vi "1122test.vi"() -> ()   [LabVIEW 2020]
uses:
  <vilib>/Instr/_visa.llb/VISA Configure Serial Port (Instr).vi
  <vilib>/Utility/file.llb/Write Delimited Spreadsheet (string).vi
panel:
  in  "文件\n路径":path=path "C:/Users/Lenovo/Desktop/data.xls"
  out "错误湿度":dbl
  out "错误温度":dbl
  out "错误芯片ID":u32
  out "温度":dbl(graph)
  out "湿度":dbl(graph)
  in  "字节数(9)":u32=9
  out "缓存区":string="23161"
  in  "串口":refnum<visa-resource-name>="COM4"
  in  "串口设置":T1={"流控制 (0:none)"=0, "停止位 (10: 1 bit)"=10, "奇偶校验 (0:none)"=0, "数据比特 (8)"=8, "比特率 (115200)"=115200} {"数据比特 (8)" min=5 max=8 step=1; "奇偶校验 (0:none)" items=["None", "Odd", "Even", "Mark", "Space"]; "流控制 (0:none)" items=["None", "XON/XOFF", "RTS/CTS", "XON/XOFF & RTS/CTS", "DTR/DSR", "XON/XOFF & DTR/DSR"]}
  in  "开关":bool=TRUE
  out "错误输出":cluster{"status":bool, i32, string}={"status"=FALSE, 1073676294, "VISA Read in Untitled 1.vi"}
  # "温湿度实时监测网络系统"
  # "设计人：苏柯宁 指导老师：李劲松"
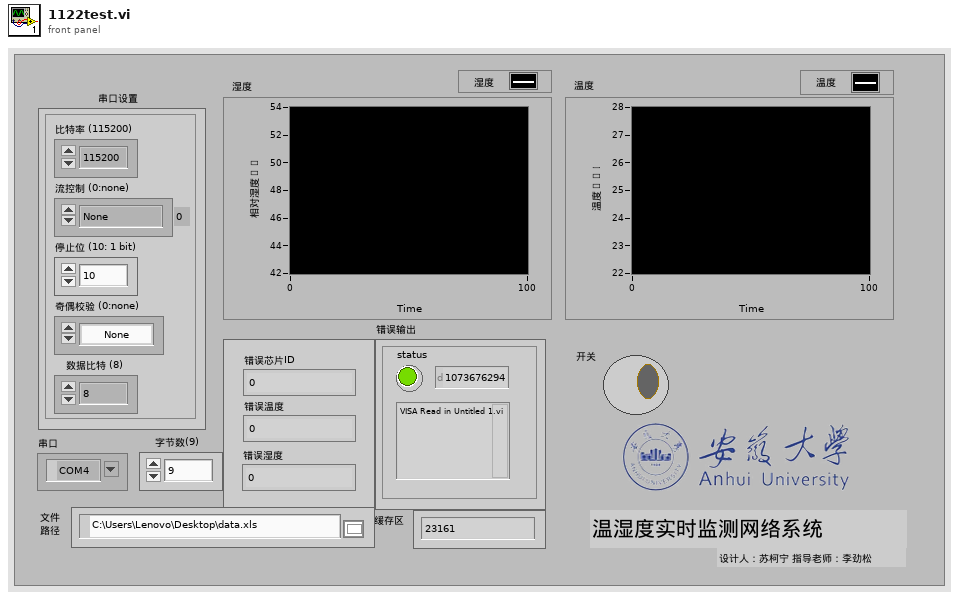
[diagram p1: front panel]
types:
  T1 = cluster{"流控制 (0:none)":u16, "停止位 (10: 1 bit)":u16, "奇偶校验 (0:none)":u16, "数据比特 (8)":u16, "比特率 (115200)":u32}
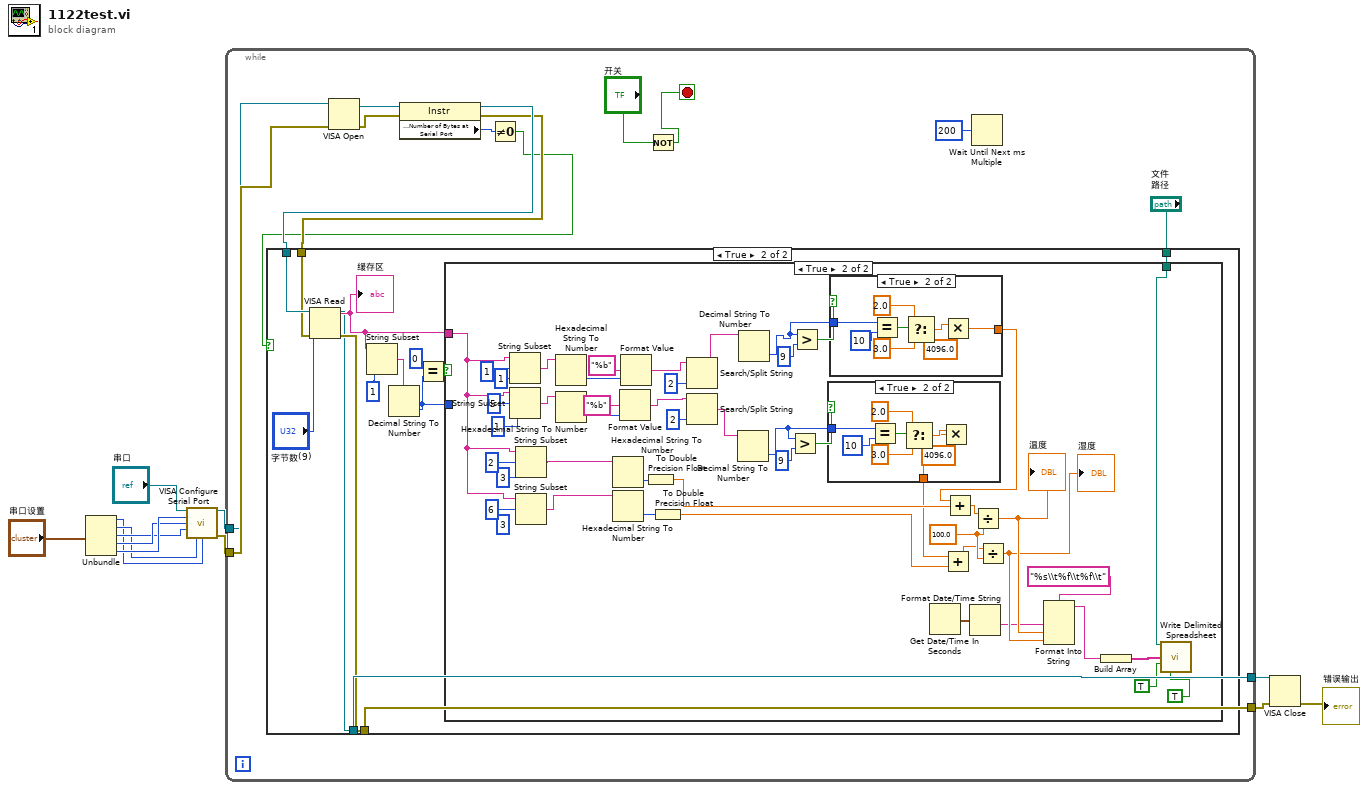
[diagram p0: block diagram]
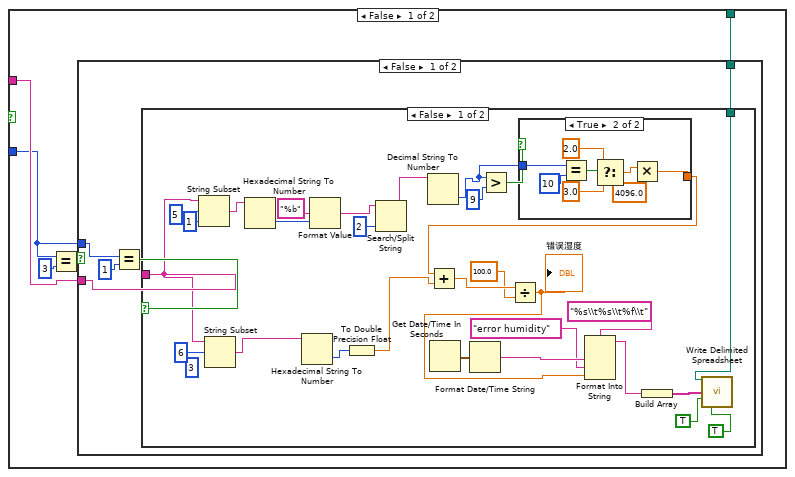
[diagram p3: hidden frame]
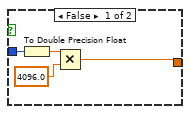
[diagram p4: hidden frame]
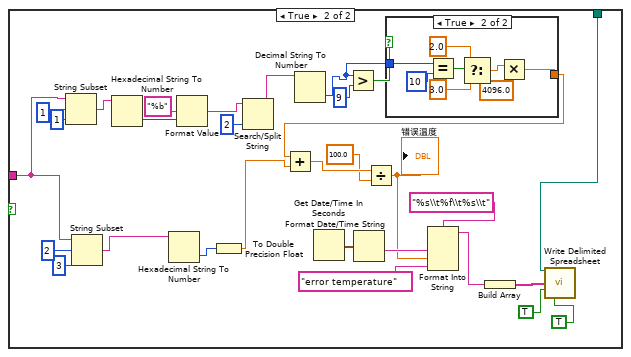
[diagram p5: hidden frame]
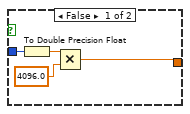
[diagram p6: hidden frame]
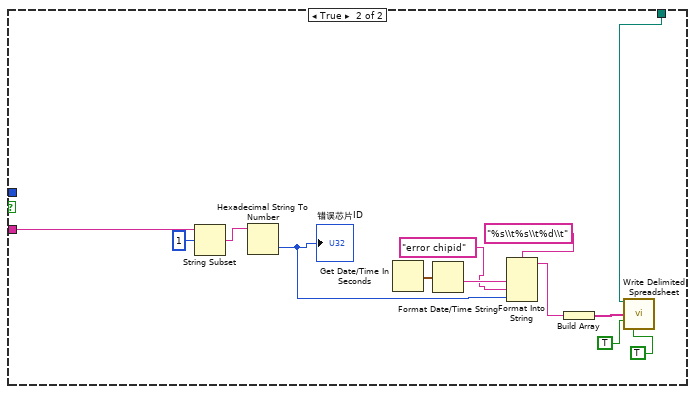
[diagram p7: hidden frame]
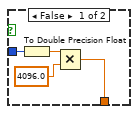
[diagram p8: hidden frame]
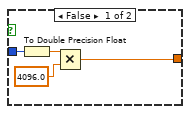
[diagram p9: hidden frame]
diagram:
  n1 = Unbundle("串口设置") -> ("流控制 (0:none)"=w6:u16, "停止位 (10: 1 bit)"=w7:u16, "奇偶校验 (0:none)"=w8:u16, "数据比特 (8)"=w9:u16, "比特率 (115200)"=w10:u32)
  n2 = call-poly "VISA Configure Serial Port"("VISA resource name"="串口", "baud rate (9600)"=w10, "data bits (8)"=w9, "parity (0:none)"=w8, "stop bits (10: 1 bit)"=w7, "flow control (0:none)"=w6) -> ("VISA resource name out"=w5:refnum<visa-resource-name>, "error out"=w4:errorcluster)  [unwired: 8 in]
  n3 = while {
    tunnel: w5 -> [w18]
    tunnel: w4 -> [w19]
    tunnel: [w26] -> w3
    tunnel: [w25] -> w2
    stop <- w13 stop-if-true
    n4 = VISA Open(error in (no error)=w19, VISA resource name=w18) -> (VISA resource name=w16:refnum<visa-resource-name>, error out=w17:errorcluster)  [unwired: 3 in]
    n5 = property class="Instr"(reference=w16, error in=w17) -> (reference out=w23:refnum<visa-resource-name>, error out=w22:errorcluster, "Serial Settings:Number of Bytes at Serial Port"=w24:u32)
    n6 = Not Equal To 0?(x=w24) -> (x != 0?=w20:bool)
    n7 = case shown="True" w20 {
      tunnel: [w28 w38] -> w26
      tunnel: [w27 w37] -> w25
      tunnel: w23 -> [w27 w36]
      tunnel: w22 -> [w28 w35]
      tunnel: "文件\n路径" -> [_ w29]
      frame False {
      }
      frame True {
        n8 = VISA Read(VISA resource name=w36, byte count="字节数(9)", error in (no error)=w35) -> (VISA resource name out=w37:refnum<visa-resource-name>, read buffer=w39:string, error out=w38:errorcluster)  [unwired: 1 out]
        "缓存区" <- w39
        n9 = String Subset(string=w39, length (rest)=1 ("length (rest)")) -> (substring=w32:string)  [unwired: 1 in]
        n10 = Decimal String To Number(string=w32) -> (number=w34:i32)  [unwired: 2 in, 1 out]
        n11 = Equal?(x=0, y=w34) -> (x = y?=w33:bool)
        n12 = case shown="True" w33 {
          tunnel: w39 -> [w43 w177]
          tunnel: w34 -> [w42 _]
          tunnel: w29 -> [w41 w147]
          frame False {
            n13 = Equal?(x=w42, y=3) -> (x = y?=w44:bool)
            n14 = case shown="False" w44 {
              tunnel: w43 -> [w47 w146]
              tunnel: w42 -> [w50 _]
              tunnel: w41 -> [w46 w134]
              frame False {
                n15 = Equal?(x=w50, y=1) -> (x = y?=w48:bool)
                n16 = case shown="False" w48 {
                  tunnel: w47 -> [w62 w104]
                  tunnel: w46 -> [w53 w94]
                  frame False {
                    (unwired) 3 ("length (rest)")
                    n17 = String Subset(string=w62, offset (0)=5, length (rest)=1 ("length (rest)")) -> (substring=w77:string)
                    n18 = String Subset(string=w62, offset (0)=6) -> (substring=w68:string)  [unwired: 1 in]
                    n19 = Hexadecimal String To Number(string=w77) -> (number=w76:u32)  [unwired: 2 in, 1 out]
                    n20 = Hexadecimal String To Number(string=w68) -> (number=w67:u32)  [unwired: 2 in, 1 out]
                    n21 = Format Value(format string="%b", value (0)=w76) -> (output string=w74:string)  [unwired: 1 in]
                    n22 = To Double Precision Float(number=w67) -> (double precision float=w66:dbl)
                    n23 = Search/Split String(string=w74, offset (0)=2) -> (match + rest of string=w71:string)  [unwired: 1 in, 2 out]
                    n24 = Decimal String To Number(string=w71) -> (number=w65:i32)  [unwired: 2 in, 1 out]
                    n25 = Get Date/Time In Seconds() -> (seconds since 1Jan1904=w56:timestamp)
                    n26 = Format Date/Time String(seconds (now)=w56) -> (date/time string=w55:string)  [unwired: 2 in]
                    n27 = Greater?(x=w65, y=9) -> (0:w69:bool)
                    n28 = case shown="True" w69 {
                      tunnel: w65 -> [w82 w91]
                      tunnel: [w80 w84] -> w63
                      frame False {
                        n29 = To Double Precision Float(number=w82) -> (double precision float=w81:dbl)
                        n30 = Multiply(x=w81, y=4096.0) -> (x*y=w80:dbl)
                      }
                      frame True {
                        n31 = Equal?(x=w91, y=10) -> (x = y?=w89:bool)
                        n32 = Select(t=2.0, s=w89, f=3.0) -> (s? t:f=w86:dbl)
                        n33 = Multiply(x=w86, y=4096.0) -> (x*y=w84:dbl)
                      }
                    }
                    n34 = Add(x=w63, y=w66) -> (x+y=w64:dbl)
                    n35 = Divide(x=w64, y=100.0) -> (x/y=w51:dbl)
                    "错误湿度" <- w51
                    n36 = Format Into String(format string="%s\\t%s\\t%f\\t", w55, "error humidity" ("input 2"), w51) -> (resulting string=w60:string)  [unwired: 2 in, 1 out]
                    n37 = Build Array(w60) -> (w59:string[])
                    n38 = call-poly <vilib>:"Write Delimited Spreadsheet.vi"("file path (dialog if empty)"=w53, "1D data"=w59, "append to file? (new file:F)"=TRUE, "transpose? (no:F)"=TRUE) -> ()  [unwired: 10 in, 2 out]
                  }
                  frame True {
                    n39 = String Subset(string=w104, offset (0)=1, length (rest)=1 ("length (rest)")) -> (substring=w119:string)
                    n40 = String Subset(string=w104, offset (0)=2, length (rest)=3 ("length (rest)")) -> (substring=w110:string)
                    n41 = Hexadecimal String To Number(string=w119) -> (number=w118:u32)  [unwired: 2 in, 1 out]
                    n42 = Hexadecimal String To Number(string=w110) -> (number=w109:u32)  [unwired: 2 in, 1 out]
                    n43 = Format Value(format string="%b", value (0)=w118) -> (output string=w116:string)  [unwired: 1 in]
                    n44 = To Double Precision Float(number=w109) -> (double precision float=w108:dbl)
                    n45 = Search/Split String(string=w116, offset (0)=2) -> (match + rest of string=w113:string)  [unwired: 1 in, 2 out]
                    n46 = Decimal String To Number(string=w113) -> (number=w107:i32)  [unwired: 2 in, 1 out]
                    n47 = Get Date/Time In Seconds() -> (seconds since 1Jan1904=w97:timestamp)
                    n48 = Greater?(x=w107, y=9) -> (0:w111:bool)
                    n49 = Format Date/Time String(seconds (now)=w97) -> (date/time string=w96:string)  [unwired: 2 in]
                    n50 = case shown="True" w111 {
                      tunnel: w107 -> [w124 w133]
                      tunnel: [w122 w126] -> w103
                      frame False {
                        n51 = To Double Precision Float(number=w124) -> (double precision float=w123:dbl)
                        n52 = Multiply(x=w123, y=4096.0) -> (x*y=w122:dbl)
                      }
                      frame True {
                        n53 = Equal?(x=w133, y=10) -> (x = y?=w131:bool)
                        n54 = Select(t=2.0, s=w131, f=3.0) -> (s? t:f=w128:dbl)
                        n55 = Multiply(x=w128, y=4096.0) -> (x*y=w126:dbl)
                      }
                    }
                    n56 = Add(x=w103, y=w108) -> (x+y=w106:dbl)
                    n57 = Divide(x=w106, y=100.0) -> (x/y=w93:dbl)
                    "错误温度" <- w93
                    n58 = Format Into String(format string="%s\\t%f\\t%s\\t", w96, w93, "error temperature" ("input 3")) -> (resulting string=w101:string)  [unwired: 2 in, 1 out]
                    n59 = Build Array(w101) -> (w100:string[])
                    n60 = call-poly <vilib>:"Write Delimited Spreadsheet.vi"("file path (dialog if empty)"=w94, "1D data"=w100, "append to file? (new file:F)"=TRUE, "transpose? (no:F)"=TRUE) -> ()  [unwired: 10 in, 2 out]
                  }
                }
              }
              frame True {
                n61 = String Subset(string=w146, offset (0)=1) -> (substring=w144:string)  [unwired: 1 in]
                n62 = Hexadecimal String To Number(string=w144) -> (number=w135:u32)  [unwired: 2 in, 1 out]
                "错误芯片ID" <- w135
                n63 = Get Date/Time In Seconds() -> (seconds since 1Jan1904=w139:timestamp)
                n64 = Format Date/Time String(seconds (now)=w139) -> (date/time string=w138:string)  [unwired: 2 in]
                n65 = Format Into String(format string="%s\\t%s\\t%d\\t", w138, "error chipid" ("input 2"), w135) -> (resulting string=w143:string)  [unwired: 2 in, 1 out]
                n66 = Build Array(w143) -> (w142:string[])
                n67 = call-poly <vilib>:"Write Delimited Spreadsheet.vi"("file path (dialog if empty)"=w134, "1D data"=w142, "append to file? (new file:F)"=TRUE, "transpose? (no:F)"=TRUE) -> ()  [unwired: 10 in, 2 out]
              }
            }
          }
          frame True {
            w154 = 100.0 ("y")
            (unwired) 3 ("length (rest)")
            n68 = String Subset(string=w177, offset (0)=1, length (rest)=1 ("length (rest)")) -> (substring=w189:string)
            n69 = String Subset(string=w177, offset (0)=5, length (rest)=1 ("length (rest)")) -> (substring=w188:string)
            n70 = String Subset(string=w177, offset (0)=2, length (rest)=3 ("length (rest)")) -> (substring=w172:string)
            n71 = String Subset(string=w177, offset (0)=6) -> (substring=w171:string)  [unwired: 1 in]
            n72 = Hexadecimal String To Number(string=w189) -> (number=w187:u32)  [unwired: 2 in, 1 out]
            n73 = Hexadecimal String To Number(string=w188) -> (number=w186:u32)  [unwired: 2 in, 1 out]
            n74 = Hexadecimal String To Number(string=w172) -> (number=w169:u32)  [unwired: 2 in, 1 out]
            n75 = Hexadecimal String To Number(string=w171) -> (number=w170:u32)  [unwired: 2 in, 1 out]
            n76 = Format Value(format string="%b", value (0)=w186) -> (output string=w180:string)  [unwired: 1 in]
            n77 = Format Value(format string="%b", value (0)=w187) -> (output string=w183:string)  [unwired: 1 in]
            n78 = To Double Precision Float(number=w169) -> (double precision float=w167:dbl)
            n79 = To Double Precision Float(number=w170) -> (double precision float=w162:dbl)
            n80 = Search/Split String(string=w183, offset (0)=2) -> (match + rest of string=w175:string)  [unwired: 1 in, 2 out]
            n81 = Search/Split String(string=w180, offset (0)=2) -> (match + rest of string=w164:string)  [unwired: 1 in, 2 out]
            n82 = Decimal String To Number(string=w164) -> (number=w160:i32)  [unwired: 2 in, 1 out]
            n83 = Decimal String To Number(string=w175) -> (number=w161:i32)  [unwired: 2 in, 1 out]
            n84 = Greater?(x=w160, y=9) -> (0:w165:bool)
            n85 = Greater?(x=w161, y=9) -> (0:w173:bool)
            n86 = case shown="True" w165 {
              tunnel: w160 -> [w196 w205]
              tunnel: [w194 w198] -> w163
              frame False {
                n87 = To Double Precision Float(number=w196) -> (double precision float=w195:dbl)
                n88 = Multiply(x=w195, y=4096.0) -> (x*y=w194:dbl)
              }
              frame True {
                n89 = Equal?(x=w205, y=10) -> (x = y?=w203:bool)
                n90 = Select(t=2.0, s=w203, f=3.0) -> (s? t:f=w200:dbl)
                n91 = Multiply(x=w200, y=4096.0) -> (x*y=w198:dbl)
              }
            }
            n92 = case shown="True" w173 {
              tunnel: w161 -> [w208 w217]
              tunnel: [w206 w210] -> w168
              frame False {
                n93 = To Double Precision Float(number=w208) -> (double precision float=w207:dbl)
                n94 = Multiply(x=w207, y=4096.0) -> (x*y=w206:dbl)
              }
              frame True {
                n95 = Equal?(x=w217, y=10) -> (x = y?=w215:bool)
                n96 = Select(t=2.0, s=w215, f=3.0) -> (s? t:f=w212:dbl)
                n97 = Multiply(x=w212, y=4096.0) -> (x*y=w210:dbl)
              }
            }
            n98 = Get Date/Time In Seconds() -> (seconds since 1Jan1904=w150:timestamp)
            n99 = Add(x=w163, y=w162) -> (x+y=w153:dbl)
            n100 = Add(x=w168, y=w167) -> (x+y=w159:dbl)
            n101 = Format Date/Time String(seconds (now)=w150) -> (date/time string=w149:string)  [unwired: 2 in]
            n102 = Divide(x=w159, y=w154) -> (x/y=w152:dbl)
            "温度" <- w152
            n103 = Divide(x=w153, y=w154) -> (x/y=w151:dbl)
            "湿度" <- w151
            n104 = Format Into String(format string="%s\\t%f\\t%f\\t", w149, w152, w151) -> (resulting string=w158:string)  [unwired: 2 in, 1 out]
            n105 = Build Array(w158) -> (w157:string[])
            n106 = call-poly <vilib>:"Write Delimited Spreadsheet.vi"("file path (dialog if empty)"=w147, "1D data"=w157, "append to file? (new file:F)"=TRUE, "transpose? (no:F)"=TRUE) -> ()  [unwired: 10 in, 2 out]
          }
        }
      }
    }
    n107 = Not(x="开关") -> (.not. x?=w13:bool)
    n108 = Wait Until Next ms Multiple(millisecond multiple=u32 200) -> ()  [unwired: 1 out]
  }
  n109 = VISA Close(VISA resource name=w2, error in (no error)=w3) -> (error out=→"错误输出":errorcluster)
